vi "Link Bus B Parameters.vi"(8 "error in (no error)":errorcluster, 11 "Bus Monitor in":refnum<class "Bus Monitor.lvclass">) -> (0 "error out":errorcluster, 3 "Bus Monitor out":refnum<class "Bus Monitor.lvclass">)   [LabVIEW 2020, in "BCI-1553 API.lvlib" / "Bus Monitor.lvclass"]
doc: "Creates a Bus Monitor-Only table of all the filters that will be operating on Bus B. This table uses command words as keys where the Word Count and Mode Code has been masked to 1F. This is used for quickly performing lookups on the current state of the monitored parameters identified in the filter. When a filter command word is not found, it remains with an unmodified value."
uses:
  Bus Monitor.lvclass
  Bus Monitor.lvclass/Bus Monitor.ctl
  Dependencies/Registry/Registry.lvclass/Registry.ctl
  Filters/Filter/Filter.lvclass
  <vilib>/Utility/error.llb/Clear Errors.vi
  Dependencies/Registry/Registry.lvclass
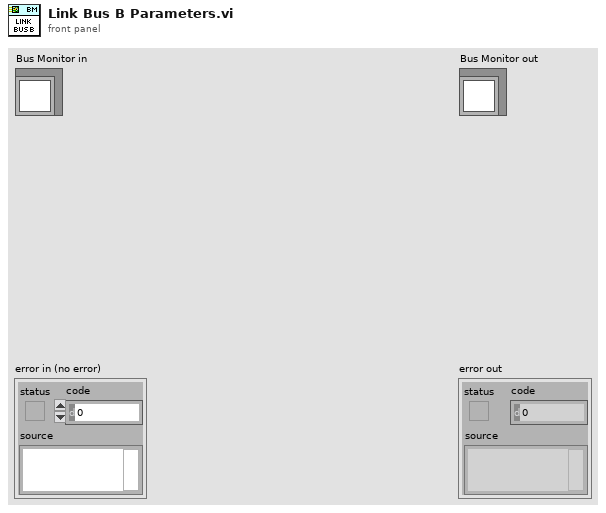
[diagram p1: front panel]
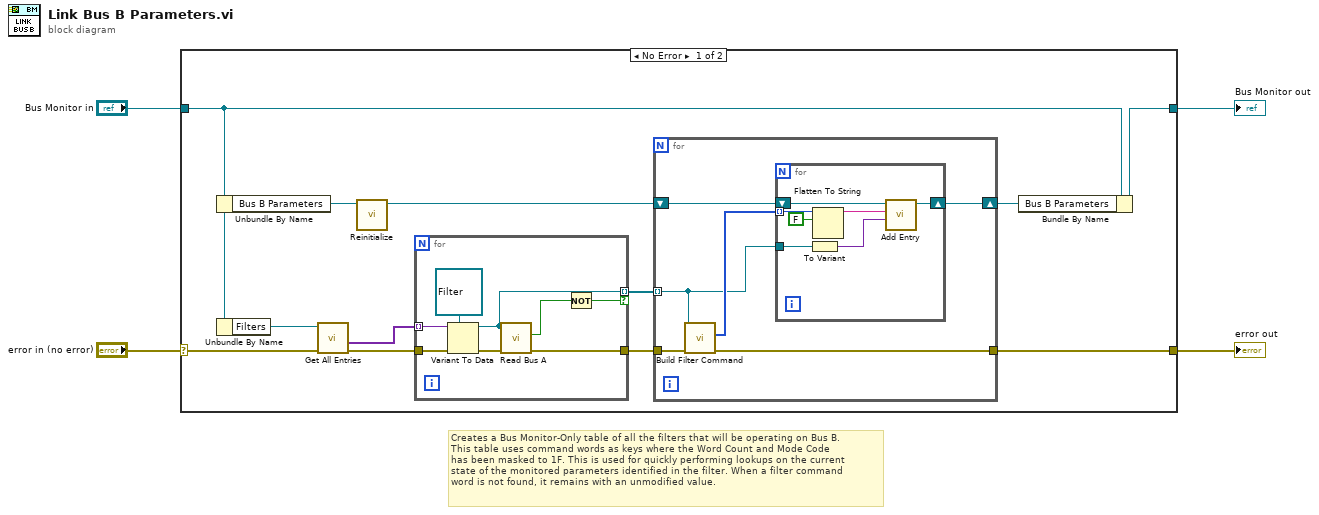
[diagram p0: block diagram]
diagram:
  # "Creates a Bus Monitor-Only table of all the filters that will be operating on Bus B.\nThis table uses command words as keys where the Word Count and Mode Code\nhas been masked to 1F. This is used for quickly performing lookups on the current\nstate of the monitored parameters identified in the filter. When a filter command\nword is not found, it remains with an unmodified value."
  n1 = case shown="No Error" "error in (no error)" {
    selector: "error in (no error)" -> [w14 w39]
    tunnel: [w10 w39] -> w1
    tunnel: [w5 w38] -> w2
    tunnel: "Bus Monitor in" -> [w6 w38]
    frame No Error {
      n2 = Unbundle By Name(w6) -> ("Bus B Parameters"=w16:refnum<class "Registry.lvclass">)
      n3 = Unbundle By Name(w6) -> ("Filters"=w15:refnum<class "Registry.lvclass">)
      n4 = call "Get All Entries.vi"("error in (no error)"=w14, "Registry in"=w15) -> ("error out"=w13:errorcluster, "Values"=w12:variant[])  [unwired: 7 in, 1 out]
      n5 = call "Reinitialize.vi"("Registry in"=w16) -> ("Registry out"=w8:refnum<class "Registry.lvclass">)  [unwired: 9 in, 1 out]
      n6 = for {
        tunnel: w12 -> [w36] mode=indexing
        tunnel: w13 -> [w34]
        tunnel: [w37] -> w11
        tunnel: [w32] -> w9 mode=indexing if=w30
        n7 = Variant To Data(error in=w34, type=refnum<class "Filter.lvclass"> refnum ("SLSC 1553 API.lvlib:Filter.lvclass"), Variant=w36) -> (data=w32:refnum<class "Filter.lvclass">, error out=w33:errorcluster)
        n8 = call-dynamic "Read Bus A.vi"("error in (no error)"=w33, "Filter in"=w32) -> ("error out"=w37:errorcluster, "Bus A?"=w31:bool)  [unwired: 7 in, 1 out]
        n9 = Not(x=w31) -> (.not. x?=w30:bool)
      }
      n10 = for {
        tunnel: w11 -> [w22]
        tunnel: [w21] -> w10
        tunnel: w9 -> [w18] mode=indexing
        shift-right: [w17] -> w7
        shift-left: w8 -> [w20]
        n11 = call-dynamic "Build Filter Command.vi"("error in (no error)"=w22, "Filter in"=w18) -> ("error out"=w21:errorcluster, "Command Words"=w19:u16[])  [unwired: 8 in]
        n12 = for {
          shift-right: [w25] -> w17
          shift-left: w20 -> [w26]
          tunnel: w19 -> [w29] mode=indexing
          tunnel: w18 -> [w27]
          n13 = To Variant(anything=w27) -> (Variant=w23:variant)
          n14 = Flatten To String(anything=w29, prepend array or string size? (T)=FALSE) -> (data string=w24:string)  [unwired: 2 in, 2 out]
          n15 = call "Add Entry.vi"("Value"=w23, "Key"=w24, "Registry in"=w26) -> ("Registry out"=w25:refnum<class "Registry.lvclass">)  [unwired: 6 in, 2 out]
        }
      }
      n16 = Bundle By Name(cluster=w6, "Bus B Parameters"=w7) -> (w5:refnum<class "Bus Monitor.lvclass">)
    }
    frame Error {
    }
  }
  "error out" <- w1
  "Bus Monitor out" <- w2
